vi "DSF.Engine.BuilderManager.Initialize Builder.vi"(7 "builder index":i32, 8 "error in (no error)":errorcluster, 10 "Framework Cache":refnum<class "DSF.Engine.Memory.Cache.Framework.lvclass">, 11 "Builder Manager in":refnum<class "DSF.Engine.BuilderManager.lvclass">) -> (0 "error out":errorcluster, 3 "Builder Manager out":refnum<class "DSF.Engine.BuilderManager.lvclass">)   [LabVIEW 2016, in "DSF.Engine.lvlib" / "DSF.Engine.BuilderManager.lvclass"]
uses:
  DSF.Engine.BuilderManager.lvclass
  Cache/DSF.Engine.Memory.Cache.Framework.lvclass
  DSF.Engine.BuilderManager.lvclass/DSF.Engine.BuilderManager.ctl
  Submodules/Memory/Source/Classes/Pointer/Memory.Pointer.lvclass/Memory.Pointer.ctl
  Submodules/Memory/Source/Classes/Pointer/Memory.Pointer.Parameter Check.Subset.vi
  Submodules/Memory/Source/Classes/Pointer/Memory.Pointer.Get Address.vi
  Submodules/Memory/Source/Classes/Pointer/Memory.Pointer.Parameter Check.Null Pointer.vi
  Submodules/Memory/Source/Classes/Pointer/Memory.Pointer.Errors.vi
  Submodules/Memory/Source/Classes/Pointer/Memory.Pointer.Errors.Out of Bounds.vi
  Submodules/Memory/Source/Classes/Pointer/Memory.Pointer.Get Size.vi
  Submodules/Memory/Source/Classes/Pointer/Memory.Pointer.Errors.Null Pointer.vi
  Submodules/Memory/Source/Submodules/SEH/Source/VIs/Static Error Handling.Source Buffer.Write.String.vi
  Submodules/Memory/Source/Classes/Pointer/Memory.Pointer.Errors.Write Pointer Size.vi
  Submodules/Memory/Source/Classes/Pointer/Memory.Pointer.Errors.Create Error.vi
  Submodules/Memory/Source/Submodules/SEH/Source/VIs/Static Error Handling.Source Buffer.Write.Numeric.Scalar.Base10.vi
  Submodules/Memory/Source/Submodules/SEH/Source/VIs/Static Error Handling.Source Buffer.Write.Numeric.Scalar.Base10 (U64).vi
  Submodules/Memory/Source/Submodules/SEH/Source/VIs/Static Error Handling.Error Cluster Constant.vi
  Submodules/Memory/Source/Submodules/SEH/Source/VIs/Static Error Handling.Error Cluster Constant (256B).vi
  Submodules/Memory/Source/Submodules/SEH/Source/VIs/Static Error Handling.Parameters.Status.Set.vi
  Submodules/Memory/Source/Submodules/SEH/Source/VIs/Static Error Handling.Parameters.Code.Set.vi
  Submodules/Memory/Source/Submodules/SEH/Source/VIs/Static Error Handling.Parameters.VI Source.Set.vi
  Submodules/Memory/Source/Constants/Memory.Constants.vi
  Submodules/Memory/Source/Constants/Memory.Constants.Library Name.vi
  Submodules/Memory/Source/Classes/Pointer/Memory.Pointer.Errors.Get Info.vi
  Status/Status.Builder.State.lvclass
  C:/Git/Sourcetree/DSF/Source/Submodules/Memory/Source/Classes/Pointer/Memory.Pointer.lvclass
  Submodules/Memory/Source/Classes/Pointer/Memory.Pointer.Encapsulate.vi
  Builder/DSF.Engine.Builder.lvclass
  Status/Status.Builder.lvclass
  Submodules/Memory/Source/Classes/Pointer/Memory.Pointer.lvclass
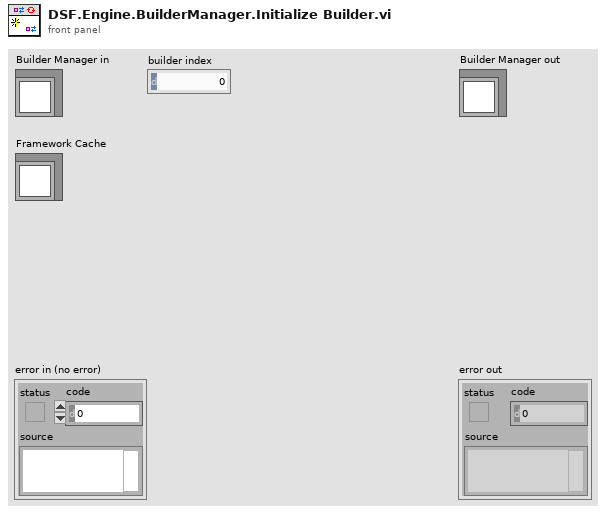
[diagram p1: front panel]
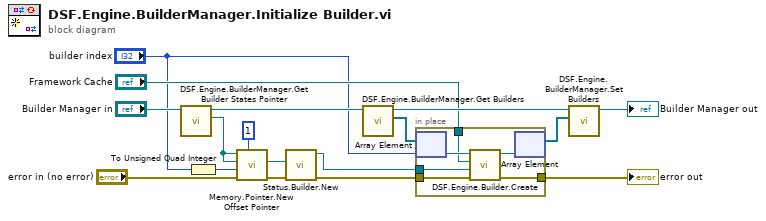
[diagram p0: block diagram]
diagram:
  n1 = call "DSF.Engine.BuilderManager.Get Builder States Pointer.vi"("Builder Manager in"="Builder Manager in") -> ("Builder States"=w14:refnum<class "Status.Builder.State.lvclass">, "Builder Manager out"=w16:refnum<class "DSF.Engine.BuilderManager.lvclass">)  [unwired: 9 in]
  n2 = To Unsigned Quad Integer(1:"builder index") -> (0:w12:u64)
  n3 = call "Memory.Pointer.New Offset Pointer.vi"("length (-1: rest)"=i64 1, "error in (no error)"="error in (no error)", "offset (0)"=w12, "offset pointer type"=w14, "base pointer in"=w14) -> ("error out"=w10:errorcluster, "offset pointer"=w11:refnum<class "Status.Builder.State.lvclass">)  [unwired: 4 in, 1 out]
  n4 = call "Status.Builder.New.vi"("error in (no error)"=w10, "Builder State Pointer"=w11) -> ("error out"=w2:errorcluster, "Builder Status"=w5:refnum<class "Status.Builder.lvclass">)  [unwired: 8 in]
  n5 = call "DSF.Engine.BuilderManager.Get Builders.vi"("Builder Manager in"=w16) -> ("Builders"=w4:refnum<class "DSF.Engine.Builder.lvclass">[], "Builder Manager out"=w9:refnum<class "DSF.Engine.BuilderManager.lvclass">)  [unwired: 9 in]
  n6 = in-place {
    in-place-border: [w21] -> w6
    in-place-border: w2 -> [w20]
    in-place-border: w5 -> [w19]
    in-place-border: "Framework Cache" -> [w18]
    n7 = in-place-array #1(w4, "builder index") -> (w23:refnum<class "DSF.Engine.Builder.lvclass">)
    n8 = call "DSF.Engine.Builder.Create.vi"("error in (no error)"=w20, "Builder Status"=w19, "Framework Cache"=w18, "Builder type"=w23) -> ("error out"=w21:errorcluster, "Builder"=w22:refnum<class "DSF.Engine.Builder.lvclass">)  [unwired: 6 in]
    n9 = in-place-array #1(w22) -> (w7:refnum<class "DSF.Engine.Builder.lvclass">[])  [unwired: 1 out]
  }
  "error out" <- w6
  n10 = call "DSF.Engine.BuilderManager.Set Builders.vi"("Builders"=w7, "Builder Manager in"=w9) -> ("Builder Manager out"=→"Builder Manager out":refnum<class "DSF.Engine.BuilderManager.lvclass">)  [unwired: 9 in]
